vi "Get XML Path.vi"(8 "error in (no error)":errorcluster, 11 "RIO Target in":refnum<class "RIO Target.lvclass">) -> (0 "error out":errorcluster, 2 "XML Path":path, 3 "RIO Target out":refnum<class "RIO Target.lvclass">)   [LabVIEW 2014, in "RIO Target.lvclass"]
uses:
  RIO Target.lvclass
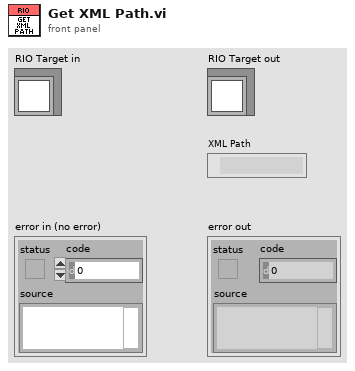
[diagram p1: front panel]
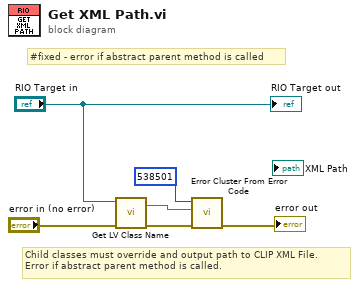
[diagram p0: block diagram]
diagram:
  # "#fixed - error if abstract parent method is called"
  # "Child classes must override and output path to CLIP XML File.\nError if abstract parent method is called."
  n1 = call <vilib>:"Get LV Class Name.vi"("error in (no error)"="error in (no error)", "object"="RIO Target in") -> ("error out"=w6:errorcluster, "class name"=w5:string)  [unwired: 8 in]
  n2 = call <vilib>:"Error Cluster From Error Code.vi"("error in (no error)"=w6, "error message (\"\")"=w5, "error code (0)"=538501) -> ("error out"=→"error out":errorcluster)  [unwired: 6 in]
  "RIO Target out" <- "RIO Target in"
